vi "momentum_chart.vi"() -> ()   [LabVIEW 2013]
uses:
  <vilib>/Utility/file.llb/Read From Spreadsheet File (DBL).vi
panel:
  out "output array":dbl[](array[numeric])
  out "subarray":dbl[](array[numeric])
  out "XY Graph":cluster{dbl[], dbl[]}[](graph)
  out "p2y":dbl[](array[numeric])
  out "p1y":dbl[](array[numeric])
  out "point frames":dbl[](array[numeric])
  out "service frames":dbl[](array[numeric])
  in  "Data file":path caption="Read data from file"
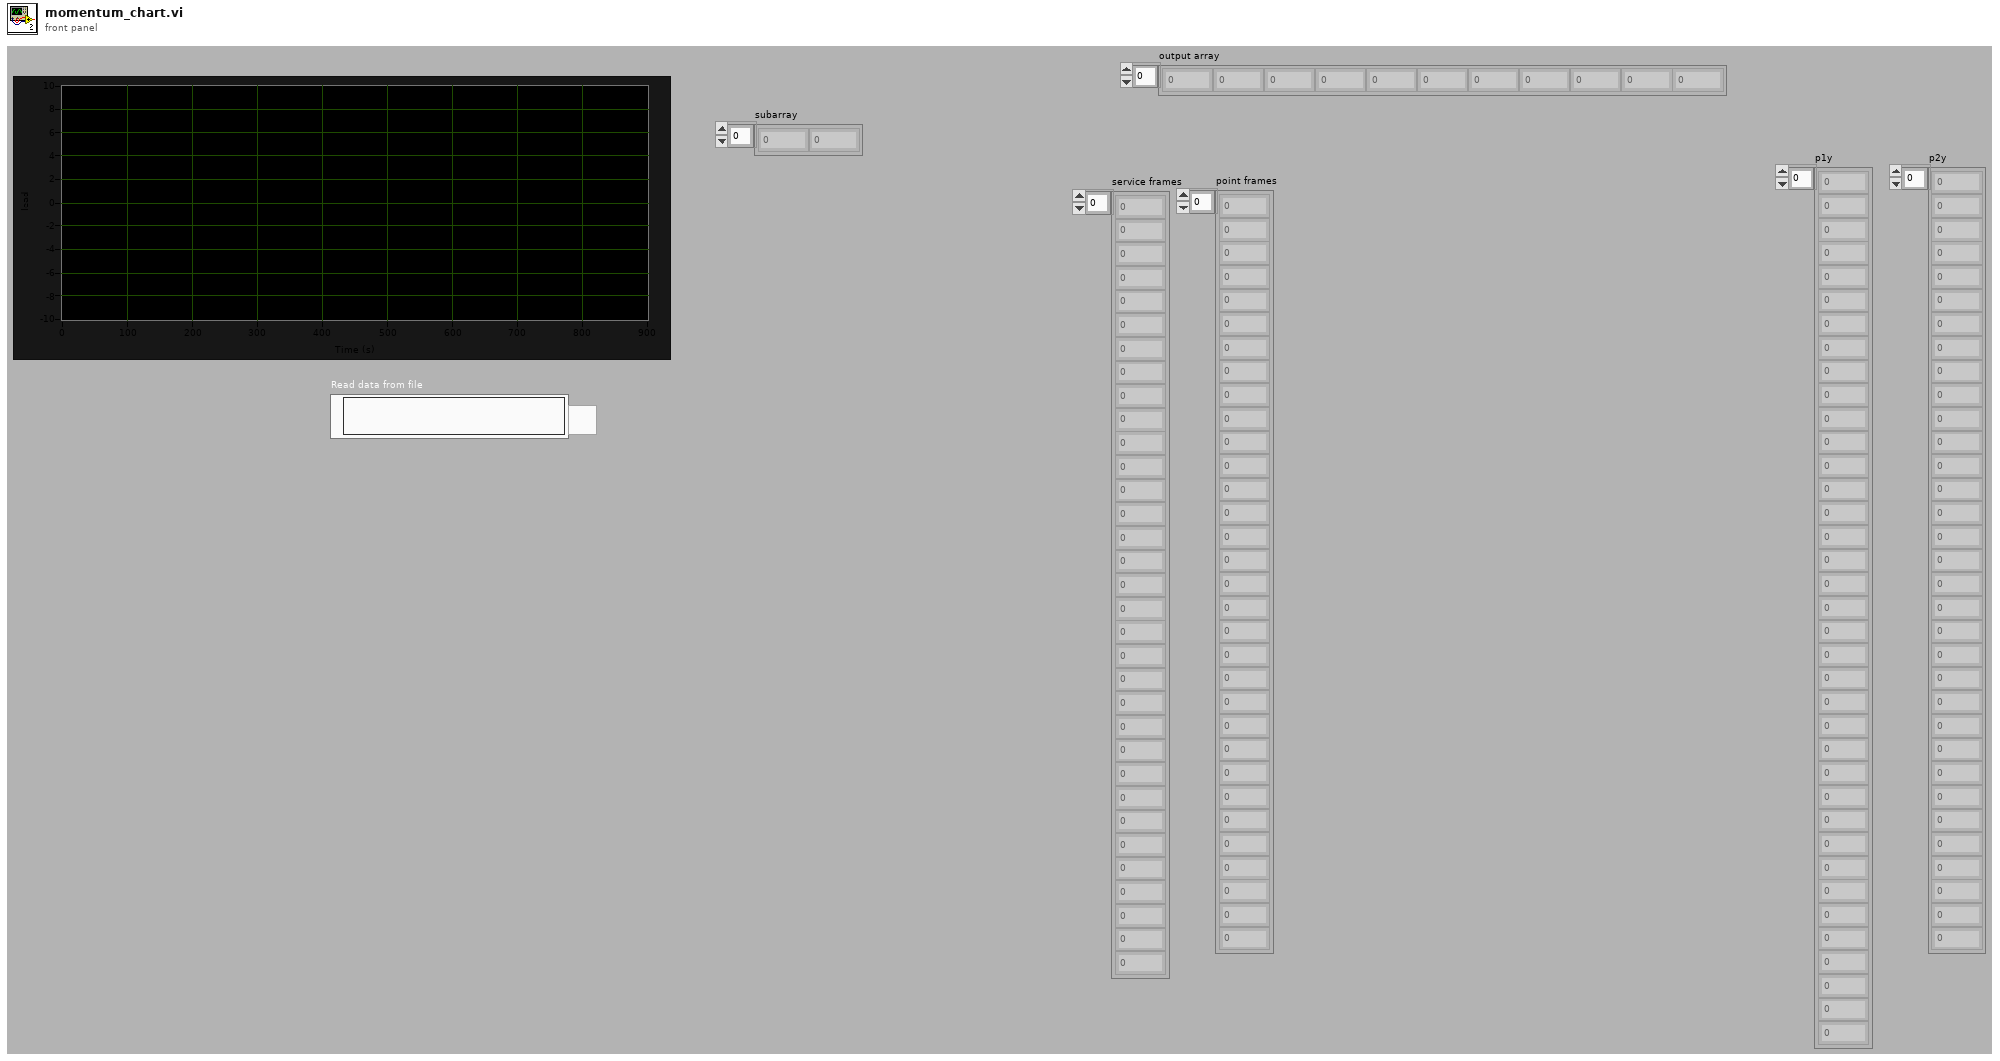
[diagram p1: front panel]
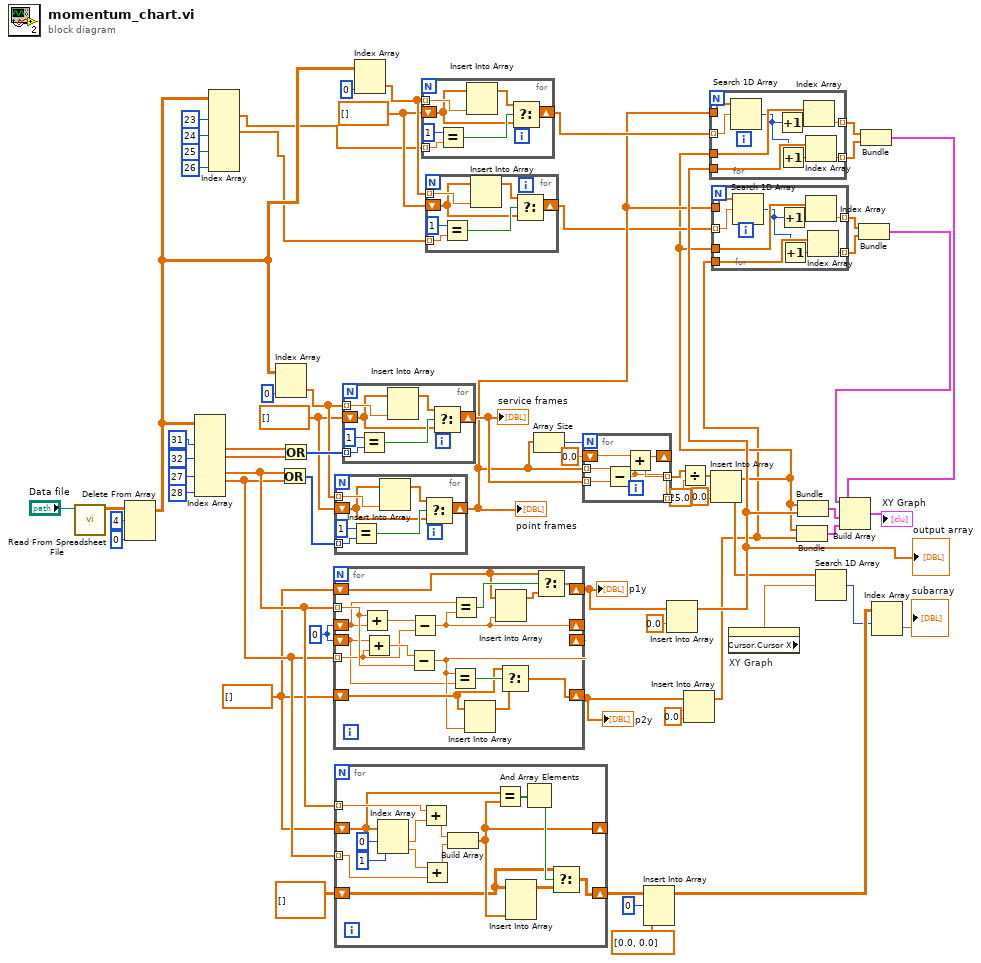
[diagram p0: block diagram]
diagram:
  w17 = dbl[] []
  w38 = 0.0 ("new element/subarray")
  w40 = 0.0 ("new element/subarray")
  w41 = 0.0 ("new element/subarray")
  w31 = dbl[] []
  w46 = 0 ("disabled index (col)")
  w49 = dbl[] []
  n1 = call-poly <vilib>:"Read From Spreadsheet File.vi"("file path (dialog if empty)"="Data file") -> ("all rows"=w60:dbl[][])  [unwired: 6 in, 4 out]
  n2 = Delete From Array(array=w60, length=4, index (row)=0) -> (array with subset deleted=w19:dbl[][])  [unwired: 1 in, 1 out]
  n3 = Index Array(array=w19, index (col) #1=31 ("length"), index (col) #2=32 ("disabled index (col)"), index (col) #3=27 ("index (col)"), index (col) #4=28 ("index (col)")) -> (element #1=w57:dbl[], element #2=w56:dbl[], element #3=w33:dbl[], element #4=w32:dbl[])  [unwired: 4 in]
  n4 = Index Array(array=w19, index (col) #1=23 ("disabled index (col)"), index (col) #2=24 ("index (col)"), index (col) #3=25 ("index (col)"), index (col) #4=26 ("index (col)")) -> (element #1=w9:dbl[], element #2=w8:dbl[])  [unwired: 4 in, 2 out]
  n5 = Index Array(array=w19, index (col)=0 ("disabled index (col)")) -> (element=w50:dbl[])  [unwired: 1 in]
  n6 = Or(x=w33, y=w32) -> (x .or. y?=w51:i32[])
  n7 = Or(x=w57, y=w56) -> (x .or. y?=w54:i32[])
  n8 = for {
    tunnel: w33 -> [w77] mode=indexing
    tunnel: w32 -> [w76] mode=indexing
    shift-right: [w68] -> _
    shift-left: w46 -> [w65]
    shift-right: [w69] -> _
    shift-left: w46 -> [w64]
    shift-right: [w66] -> w37
    shift-left: w31 -> [w67]
    shift-right: [w73] -> w39
    shift-left: w31 -> [w74]
    n9 = Add(x=w77, y=w65) -> (x+y=w78:dbl)
    n10 = Add(x=w64, y=w76) -> (x+y=w79:dbl)
    n11 = Subtract(x=w79, y=w77) -> (x-y=w69:dbl)
    n12 = Subtract(x=w78, y=w76) -> (x-y=w68:dbl)
    n13 = Equal?(x=w69, y=w64) -> (x = y?=w75:bool)
    n14 = Equal?(x=w65, y=w68) -> (x = y?=w72:bool)
    n15 = Insert Into Array(array=w74, new element=w69) -> (w70:dbl[])  [unwired: 1 in]
    n16 = Insert Into Array(array=w67, new element=w68) -> (w71:dbl[])  [unwired: 1 in]
    n17 = Select(t=w74, s=w75, f=w70) -> (s? t:f=w73:dbl[])
    n18 = Select(t=w67, s=w72, f=w71) -> (s? t:f=w66:dbl[])
  }
  "p1y" <- w37
  "p2y" <- w39
  n19 = for {
    tunnel: w51 -> [w86] mode=indexing
    tunnel: w50 -> [w82] mode=indexing
    shift-right: [w81] -> w7
    shift-left: w49 -> [w80]
    n20 = Equal?(x=1, y=w86) -> (x = y?=w84:bool)
    n21 = Insert Into Array(array=w80, new element=w82) -> (w83:dbl[])  [unwired: 1 in]
    n22 = Select(t=w83, s=w84, f=w80) -> (s? t:f=w81:dbl[])
  }
  "point frames" <- w7
  n23 = for {
    tunnel: w33 -> [w98] mode=indexing
    tunnel: w32 -> [w94] mode=indexing
    shift-right: [w90] -> _
    shift-left: w31 -> [w93]
    shift-right: [w88] -> w29
    shift-left: dbl[][] [] -> [w87]
    n24 = Index Array(array=w93, index #1=0 ("index"), index #2=1 ("index")) -> (element #1=w99:dbl, element #2=w97:dbl)
    n25 = Add(x=w98, y=w99) -> (x+y=w96:dbl)
    n26 = Add(x=w97, y=w94) -> (x+y=w95:dbl)
    n27 = Build Array(w96, w95) -> (w90:dbl[])
    n28 = Equal?(x=w93, y=w90) -> (x = y?=w92:bool[])
    n29 = Insert Into Array(array=w87, new element=w90) -> (w89:dbl[][])  [unwired: 2 in]
    n30 = And Array Elements(Boolean array=w92) -> (logical AND=w91:bool)
    n31 = Select(t=w87, s=w91, f=w89) -> (s? t:f=w88:dbl[][])
  }
  n32 = for {
    tunnel: w54 -> [w108] mode=indexing
    tunnel: w50 -> [w104] mode=indexing
    shift-right: [w103] -> w47
    shift-left: w49 -> [w102]
    n33 = Equal?(x=1, y=w108) -> (x = y?=w106:bool)
    n34 = Insert Into Array(array=w102, new element=w104) -> (w105:dbl[])  [unwired: 1 in]
    n35 = Select(t=w105, s=w106, f=w102) -> (s? t:f=w103:dbl[])
  }
  "service frames" <- w47
  n36 = Index Array(array=w19, index (col)=0 ("disabled index (col)")) -> (element=w18:dbl[])  [unwired: 1 in]
  n37 = for {
    tunnel: w9 -> [w115] mode=indexing
    tunnel: w18 -> [w111] mode=indexing
    shift-right: [w110] -> w14
    shift-left: w17 -> [w109]
    n38 = Equal?(x=1, y=w115) -> (x = y?=w113:bool)
    n39 = Insert Into Array(array=w109, new element=w111) -> (w112:dbl[])  [unwired: 1 in]
    n40 = Select(t=w112, s=w113, f=w109) -> (s? t:f=w110:dbl[])
  }
  n41 = for {
    tunnel: w8 -> [w122] mode=indexing
    tunnel: w18 -> [w118] mode=indexing
    shift-right: [w117] -> w6
    shift-left: w17 -> [w116]
    n42 = Equal?(x=1, y=w122) -> (x = y?=w120:bool)
    n43 = Insert Into Array(array=w116, new element=w118) -> (w119:dbl[])  [unwired: 1 in]
    n44 = Select(t=w119, s=w120, f=w116) -> (s? t:f=w117:dbl[])
  }
  n45 = Array Size(array=w7) -> (size(s)=w48:i32)
  n46 = for {
    N: w48 -> [_]
    tunnel: w7 -> [w127] mode=indexing
    tunnel: w47 -> [w126] mode=indexing
    tunnel: [w124] -> w35 mode=indexing
    shift-right: [w124] -> _
    shift-left: 0.0 -> [w125]
    tunnel: [w123] -> _ mode=indexing
    n47 = Subtract(x=w127, y=w126) -> (x-y=w123:dbl)
    n48 = Add(x=w125, y=w123) -> (x+y=w124:dbl)
  }
  n49 = Insert Into Array(array=w29, index (row)=0, new element=dbl[] [0.0, 0.0] ("new element/subarray")) -> (w25:dbl[][])  [unwired: 1 in]
  n50 = Insert Into Array(array=w37, index=w38, new element=w38) -> (w13:dbl[])
  "output array" <- w13
  n51 = Divide(x=w35, y=25.0 ("new element/subarray")) -> (x/y=w36:dbl[])
  n52 = Insert Into Array(array=w39, index=w40, new element=w40) -> (w4:dbl[])
  n53 = Insert Into Array(array=w36, index=w41, new element=w41) -> (w5:dbl[])
  n54 = for {
    tunnel: w14 -> [w136] mode=indexing
    tunnel: w7 -> [w135]
    tunnel: w5 -> [w134]
    tunnel: [w132] -> w12 mode=indexing
    tunnel: w13 -> [w130]
    tunnel: [w128] -> w11 mode=indexing
    n55 = Search 1D Array(1D array=w135, element=w136) -> (index of element=w129:i32)  [unwired: 1 in]
    n56 = Increment(x=w129) -> (x+1=w133:i32)
    n57 = Increment(x=w129) -> (x+1=w131:i32)
    n58 = Index Array(array=w134, index=w133) -> (element=w132:dbl)
    n59 = Index Array(array=w130, index=w131) -> (element=w128:dbl)
  }
  n60 = for {
    tunnel: w6 -> [w145] mode=indexing
    tunnel: w7 -> [w144]
    tunnel: w5 -> [w143]
    tunnel: [w141] -> w3 mode=indexing
    tunnel: w4 -> [w139]
    tunnel: [w137] -> w2 mode=indexing
    n61 = Search 1D Array(1D array=w144, element=w145) -> (index of element=w138:i32)  [unwired: 1 in]
    n62 = Increment(x=w138) -> (x+1=w142:i32)
    n63 = Increment(x=w138) -> (x+1=w140:i32)
    n64 = Index Array(array=w143, index=w142) -> (element=w141:dbl)
    n65 = Index Array(array=w139, index=w140) -> (element=w137:dbl)
  }
  n66 = property on="XY Graph" class="XYGraph (strict)"() -> ("Cursor.Cursor X"=w26:dbl)  [unwired: 2 in, 2 out]
  n67 = Bundle(w5, w4) -> (w45:cluster{dbl[], dbl[]})  [unwired: 1 in]
  n68 = Bundle(w5, w13) -> (w44:cluster{dbl[], dbl[]})  [unwired: 1 in]
  n69 = Search 1D Array(1D array=w5, element=w26) -> (index of element=w24:i32)  [unwired: 1 in]
  n70 = Bundle(w3, w2) -> (w1:cluster{dbl[], dbl[]})  [unwired: 1 in]
  n71 = Bundle(w12, w11) -> (w10:cluster{dbl[], dbl[]})  [unwired: 1 in]
  n72 = Build Array(w1, w10, w44, w45) -> (→"XY Graph":cluster{dbl[], dbl[]}[])
  n73 = Index Array(array=w25, index (row)=w24) -> (element=→"subarray":dbl[])  [unwired: 1 in]
